vi "Configure Multipoint.vi"(8 "error in (no error)":errorcluster, 9 "Sample Count (1)":i32=1 format="%#.6g", 10 "Trigger Count (1)":i32=1 format="%#.6g", 11 "VISA resource name":refnum<visa-resource-name>) -> (0 "error out":errorcluster, 3 "VISA resource name out":refnum<visa-resource-name>)   [LabVIEW 2020, in "PICOTEST M351XA Series.lvlib"]
doc: "Configures trigger count and sample count so you can take multipoint measurements.\n\nNote: Use this VI only with other low-level VIs. The high-level VIs automatically incorporate this functionality."
uses:
  PICOTEST M351XA Series.lvlib
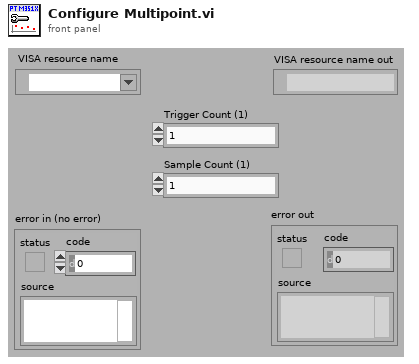
[diagram p1: front panel]
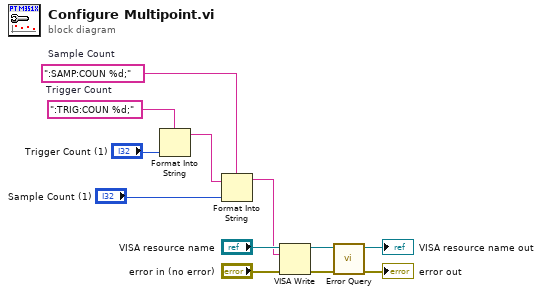
[diagram p0: block diagram]
diagram:
  w4 = ":SAMP:COUN %d;"  # Sample Count
  w5 = ":TRIG:COUN %d;"  # Trigger Count
  n1 = Format Into String(format string=w5, "Trigger Count (1)") -> (resulting string=w2:string)  [unwired: 2 in, 1 out]
  n2 = Format Into String(format string=w4, initial string=w2, "Sample Count (1)") -> (resulting string=w1:string)  [unwired: 1 in, 1 out]
  n3 = VISA Write(VISA resource name="VISA resource name", write buffer=w1, error in (no error)="error in (no error)") -> (VISA resource name out=w8:refnum<visa-resource-name>, error out=w7:errorcluster)  [unwired: 1 out]
  n4 = call "Error Query.vi"("error in (no error)"=w7, "VISA resource name"=w8) -> ("error out"=→"error out":errorcluster, "VISA resource name out"=→"VISA resource name out":refnum<visa-resource-name>)  [unwired: 6 in, 2 out]
